vi "QA_500.vi"(8 "ERRIN":errorcluster caption="entrée d'erreur (pas d'erreur)", 10 "VISA":refnum<visa-resource-name>) -> (0 "ERROUT":errorcluster caption="sortie d'erreur", 2 "DATAOUT":string)   [LabVIEW 2020]
panel:
  # "<\\B20\\BE:(A\\CC\\A9:P\\D2\\C5SS\\C9\\CFN\\A0HAU\\D4\\C5\\8D\\n"
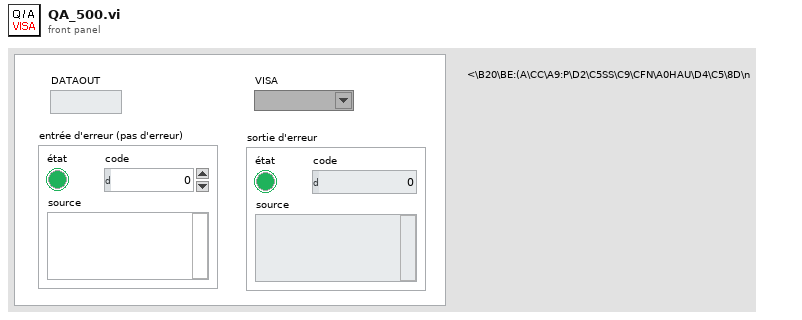
[diagram p1: front panel]
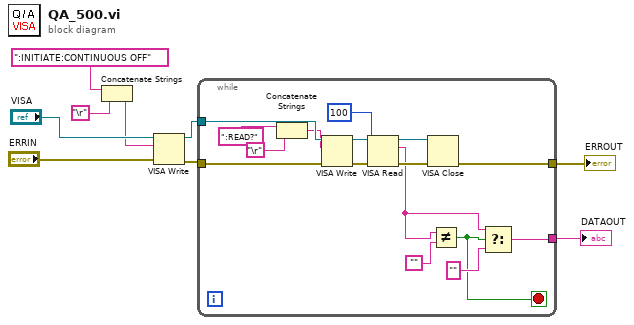
[diagram p0: block diagram]
diagram:
  n1 = Concatenate Strings(":INITIATE:CONTINUOUS OFF", "\r") -> (w3:string)
  n2 = VISA Write(VISA resource name="VISA", write buffer=w3, error in (no error)="ERRIN") -> (VISA resource name out=w2:refnum<visa-resource-name>, error out=w1:errorcluster)  [unwired: 1 out]
  n3 = while {
    tunnel: [w25] -> w9
    tunnel: [w24] -> w8
    tunnel: w1 -> [w14]
    tunnel: w2 -> [w13]
    stop <- w15 stop-if-true
    n4 = Concatenate Strings(":READ?", "\r") -> (w10:string)
    n5 = VISA Write(VISA resource name=w13, write buffer=w10, error in (no error)=w14) -> (VISA resource name out=w19:refnum<visa-resource-name>, error out=w21:errorcluster)  [unwired: 1 out]
    n6 = VISA Read(VISA resource name=w19, byte count=u32 100 ("nombre d'octets"), error in (no error)=w21) -> (VISA resource name out=w22:refnum<visa-resource-name>, read buffer=w16:string, error out=w23:errorcluster)  [unwired: 1 out]
    n7 = VISA Close(VISA resource name=w22, error in (no error)=w23) -> (error out=w25:errorcluster)
    n8 = Not Equal?(x=w16, y="") -> (x != y?=w15:bool)
    n9 = Select(t=w16, s=w15, f="") -> (s? t:f=w24:string)
  }
  "ERROUT" <- w9
  "DATAOUT" <- w8
